vi "Calculate_Distance.vi"(8 "error in (no error)":errorcluster, 9 "B":cluster{"X":dbl, "Y":dbl}, 10 "A":cluster{"X":dbl, "Y":dbl}) -> (0 "error out":errorcluster, 2 "Distance":dbl)   [LabVIEW 2018]
doc: "Calculates the distance between two points (position and destination) by using the distance formula."
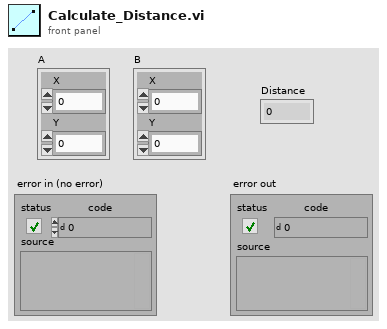
[diagram p1: front panel]
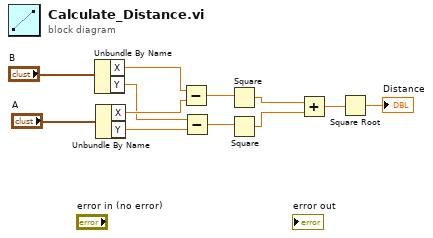
[diagram p0: block diagram]
diagram:
  n1 = Unbundle By Name("B") -> ("X"=w10:dbl, "Y"=w8:dbl)
  n2 = Unbundle By Name("A") -> ("X"=w9:dbl, "Y"=w7:dbl)
  n3 = Subtract(x=w10, y=w9) -> (x-y=w5:dbl)
  n4 = Subtract(x=w8, y=w7) -> (x-y=w6:dbl)
  n5 = Square(x=w5) -> (x^2=w4:dbl)
  n6 = Square(x=w6) -> (x^2=w3:dbl)
  n7 = Add(x=w4, y=w3) -> (x+y=w2:dbl)
  n8 = Square Root(x=w2) -> (sqrt(x)=→"Distance":dbl)
